vi "Init.vi"(8 "error in (no error)":errorcluster, 10 "Serial Config":T1={"Com Port"="", "baud rate"=0, "data bits"=8, "parity"=enum."None", "stop bits"=0, "flow control "=0, "timeout "=10000} {"data bits" min=5 max=8 step=1; "flow control" items=["None", "XON/XOFF", "RTS/CTS", "XON/XOFF & RTS/CTS", "DTR/DSR", "XON/XOFF & DTR/DSR"]}, 11 "Serial Base in":refnum<class "Serial Base.lvclass">) -> (0 "error out":errorcluster, 3 "Serial Base out":refnum<class "Serial Base.lvclass">)   [LabVIEW 2014, in "Serial Base.lvclass"]
uses:
  Serial Base.lvclass
  Object Argument--cluster.ctl
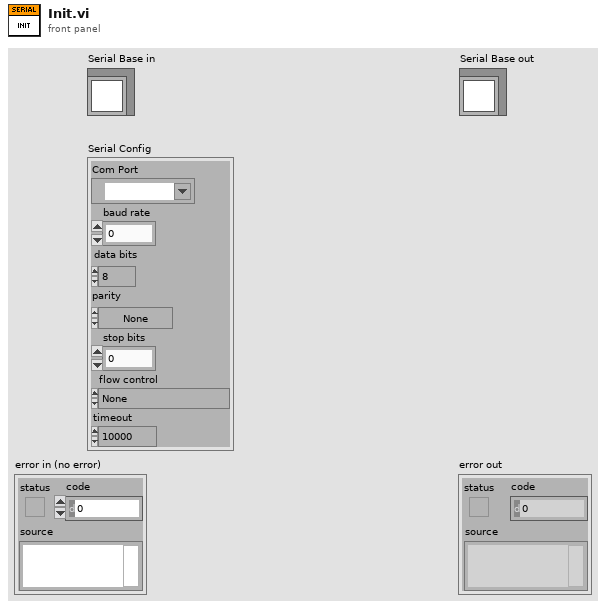
[diagram p1: front panel]
types:
  T1 = typedef "Serial Base.lvclass/Object Argument--cluster.ctl" = cluster{"Com Port":refnum<visa-resource-name>, "baud rate":u32, "data bits":u16, "parity":enum16{"None", "Odd", "Even", "Mark", "Space"}, "stop bits":u16, "flow control ":u16, "timeout ":u32}
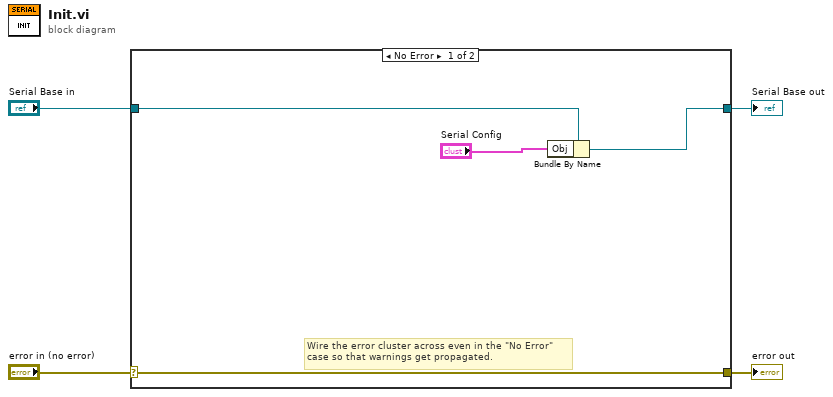
[diagram p0: block diagram]
diagram:
  n1 = case shown="No Error" "error in (no error)" {
    selector: "error in (no error)" -> [w8 w10]
    tunnel: [w8 w10] -> w3
    tunnel: [w6 w9] -> w1
    tunnel: "Serial Base in" -> [w7 w9]
    frame No Error {
      # "Wire the error cluster across even in the \"No Error\"\ncase so that warnings get propagated."
      n2 = Bundle By Name(cluster=w7, "Obj"="Serial Config") -> (w6:refnum<class "Serial Base.lvclass">)
    }
    frame Error {
    }
  }
  "error out" <- w3
  "Serial Base out" <- w1
